vi "Construct.vi"(8 "error in (no error)":errorcluster, 11 "id":string) -> (0 "error out":errorcluster, 3 "Execution Unit Implementation":refnum<class "Execution Unit.lvclass">)   [LabVIEW 2020, in "Ballard ARINC 429 Engine.lvlib" / "Implementation.lvlib" / "Execution Unit.lvclass"]
uses:
  Execution Unit.lvclass
  Execution Unit.lvclass/Execution Unit.ctl
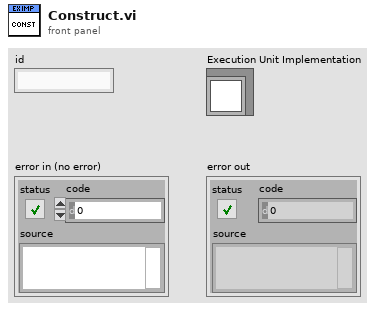
[diagram p1: front panel]
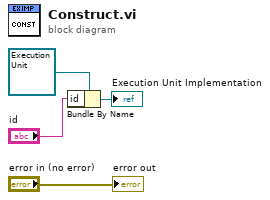
[diagram p0: block diagram]
diagram:
  n1 = Bundle By Name(cluster=refnum<class "Execution Unit.lvclass"> refnum ("Execution Unit Implementation"), "id"="id") -> (→"Execution Unit Implementation":refnum<class "Execution Unit.lvclass">)
  "error out" <- "error in (no error)"
